vi "Convert To JSON Comp Format.vi"(11 "input settings":T2={"number of channels"=51200, "data justification"=enum."Right Justified", "endianness"=enum."MSB First", "channel length"=0, "bit depth"=0, "frame clock rate"=0.0, "bit clock edge sync"=enum."Falling", "master clock source"=enum."Internal", "master clock rate"=0.0, "Logic Level"=enum."1.2 V", "frame sync edge for channel 0"=enum."Rising", "Channel 0 Offset"=0}) -> (3 "input settings JSON":cluster{"digital serial":T1})   [LabVIEW 2022 SP3, in "digital serial input cfg file.lvlib"]
uses:
  digital serial input cfg file.lvlib
  controls/digital serial audio/digital serial input settings.ctl
  <vilib>/PDM Acquisition Toolkit/shared/controls/PCM Data Justification.ctl
  <vilib>/PDM Acquisition Toolkit/shared/controls/PCM Bit Endianness.ctl
  <vilib>/PDM Acquisition Toolkit/shared/controls/Digital Edge.ctl
  controls/master clock source.ctl
  <vilib>/PDM Acquisition Toolkit/host/Classes/Session/Controls/Logic Levels.ctl
  controls/digital serial audio/digital serial input settings_json.ctl
  <vilib>/PDM Acquisition Toolkit/shared/PDM Shared.lvlib
  <vilib>/PDM Acquisition Toolkit/host/Classes/Session/DecoderSession.lvclass
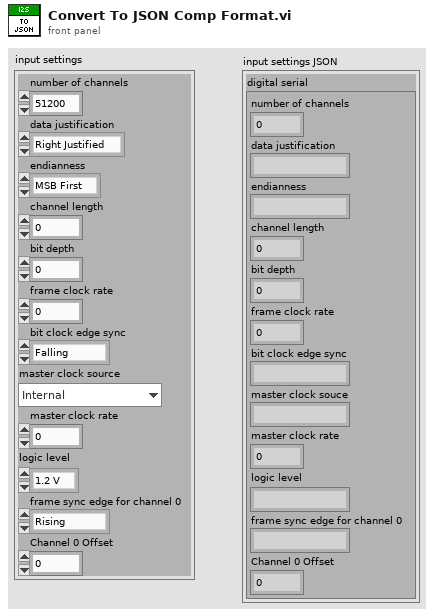
[diagram p1: front panel]
types:
  T1 = typedef "digital serial input settings_json.ctl" = cluster{"number of channels":u32, "data justification":string, "endianness":string, "channel length":u32, "bit depth":u32, "frame clock rate":dbl, "bit clock edge sync":string, "master clock souce":string, "master clock rate":dbl, "logic level":string, "frame sync edge for channel 0":string, "Channel 0 Offset":u32}
  T2 = typedef "digital serial input settings.ctl" = cluster{"number of channels":u32, "data justification":T3, "endianness":T4, "channel length":u32, "bit depth":u32, "frame clock rate":dbl, "bit clock edge sync":T5, "master clock source":T6, "master clock rate":dbl, "Logic Level":T7, "frame sync edge for channel 0":T5, "Channel 0 Offset":u32}
  T3 = typedef "PDM Shared.lvlib/PCM Data Justification.ctl" = enum16{"Left Justified", "Right Justified"}
  T4 = typedef "PDM Shared.lvlib/PCM Bit Endianness.ctl" = enum16{"MSB First", "LSB First"}
  T5 = typedef "PDM Shared.lvlib/Digital Edge.ctl" = enum8{"Rising", "Falling"}
  T6 = typedef "master clock source.ctl" = enum32{"Internal", "External"}
  T7 = typedef "PDM Acquisition Class Library.lvlib/DecoderSession.lvclass/Logic Levels.ctl" = enum16{"3.3 V", "1.8 V", "1.2 V"}
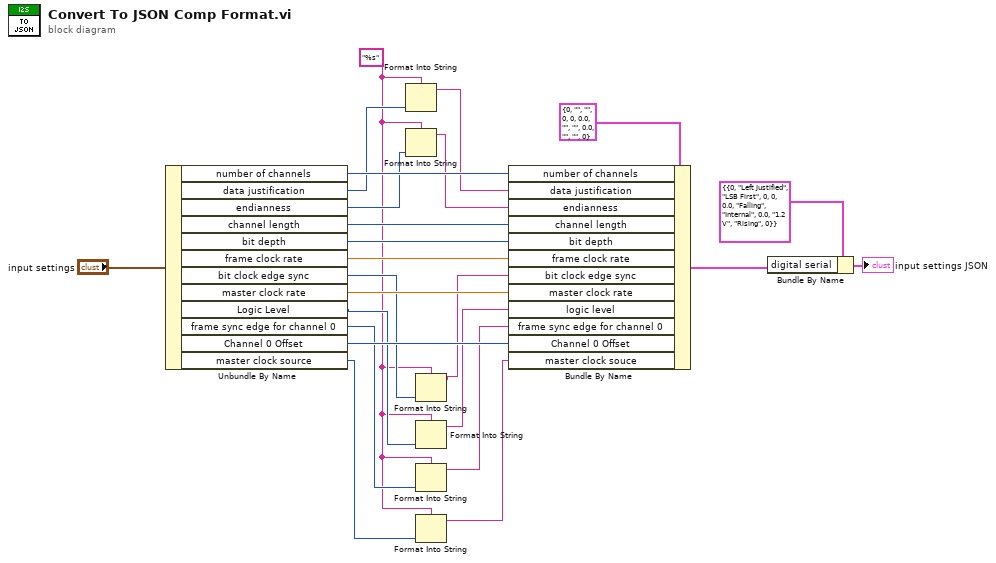
[diagram p0: block diagram]
diagram:
  w6 = "%s" ("format string")
  n1 = Unbundle By Name("input settings") -> ("number of channels"=w23:u32, "data justification"=w17:T3, "endianness"=w15:T4, "channel length"=w22:u32, "bit depth"=w21:u32, "frame clock rate"=w20:dbl, "bit clock edge sync"=w13:T5, "master clock rate"=w19:dbl, "Logic Level"=w12:T7, "frame sync edge for channel 0"=w11:T5, "Channel 0 Offset"=w18:u32, "master clock source"=w7:T6)
  n2 = Format Into String(format string=w6, w17) -> (resulting string=w16:string)  [unwired: 2 in, 1 out]
  n3 = Format Into String(format string=w6, w15) -> (resulting string=w14:string)  [unwired: 2 in, 1 out]
  n4 = Format Into String(format string=w6, w13) -> (resulting string=w9:string)  [unwired: 2 in, 1 out]
  n5 = Format Into String(format string=w6, w12) -> (resulting string=w8:string)  [unwired: 2 in, 1 out]
  n6 = Format Into String(format string=w6, w11) -> (resulting string=w10:string)  [unwired: 2 in, 1 out]
  n7 = Format Into String(format string=w6, w7) -> (resulting string=w5:string)  [unwired: 2 in, 1 out]
  n8 = Bundle By Name(cluster=T1 {"number of channels"=0, "data justification"="", "endianness"="", "channel length"=0, "bit depth"=0, "frame clock rate"=0.0, "bit clock edge sync"="", "master clock souce"="", "master clock rate"=0.0, "logic level"="", "frame sync edge for channel 0"="", "Channel 0 Offset"=0} ("JSON compatible settings"), "number of channels"=w23, "data justification"=w16, "endianness"=w14, "channel length"=w22, "bit depth"=w21, "frame clock rate"=w20, "bit clock edge sync"=w9, "master clock rate"=w19, "logic level"=w8, "frame sync edge for channel 0"=w10, "Channel 0 Offset"=w18, "master clock souce"=w5) -> (w2:T1)
  n9 = Bundle By Name(cluster=cluster{"digital serial":T1} {"digital serial"={"number of channels"=0, "data justification"="Left Justified", "endianness"="LSB First", "channel length"=0, "bit depth"=0, "frame clock rate"=0.0, "bit clock edge sync"="Falling", "master clock souce"="Internal", "master clock rate"=0.0, "logic level"="1.2 V", "frame sync edge for channel 0"="Rising", "Channel 0 Offset"=0}}, "digital serial"=w2) -> (→"input settings JSON":cluster{"digital serial":T1})
